vi "remove node name.vi"(8 "error in (no error)":errorcluster, 11 "Data Value Reference in":refnum<data-value>) -> (0 "error out":errorcluster, 3 "Data Value Reference out":refnum<data-value>, 5 "nodes alive":string[](array[string]))   [LabVIEW 2020, in "Publisher Subscriber.lvlib"]
uses:
  Publisher Subscriber.lvlib
  Controls/node dvr data.ctl
  Controls/data cluster.ctl
  Controls/subscription bank ref.ctl
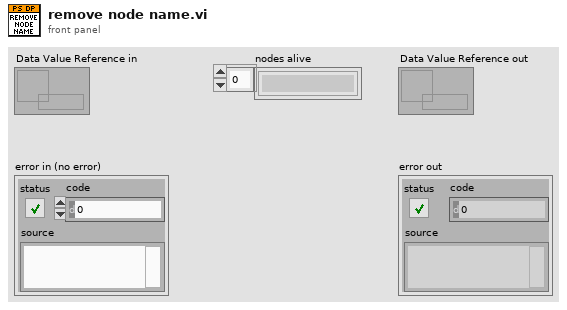
[diagram p1: front panel]
types:
  T1 = typedef "Publisher Subscriber.lvlib/node dvr data.ctl" = cluster{"queue ref":refnum<queue>, "Subscription Bank Ref":refnum<data-value>, "Command":string, "Data":variant, "Subscriptions []":set{string}, "Variables DVR Ref":refnum<data-value>}
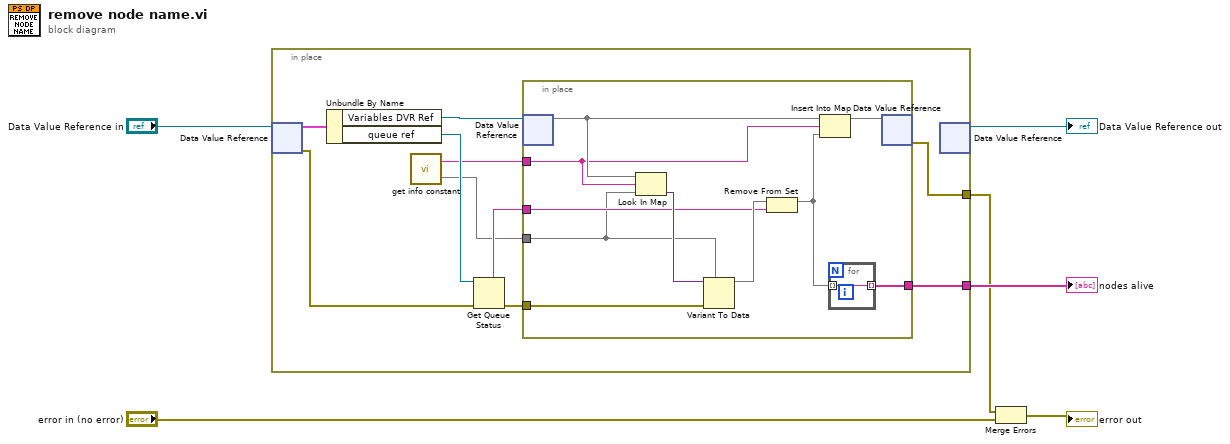
[diagram p0: block diagram]
diagram:
  n1 = in-place {
    in-place-border: [w11] -> w3
    in-place-border: [w10] -> w4
    n2 = in-place-dvr #1("Data Value Reference in") -> (w16:T1, w9:errorcluster)
    n3 = Unbundle By Name(w16) -> ("Variables DVR Ref"=w15:refnum<data-value>, "queue ref"=w14:refnum<queue>)
    n4 = call "get info constant.vi"() -> ("set"=w7:set{string}, "String"=w8:string)  [unwired: 4 in]
    n5 = Get Queue Status(queue=w14, error in (no error)=w9) -> (queue name=w13:string, error out=w12:errorcluster)  [unwired: 1 in, 6 out]
    n6 = in-place {
      in-place-border: w13 -> [w23]
      in-place-border: w8 -> [w22]
      in-place-border: w12 -> [w20]
      in-place-border: [w19] -> w10
      in-place-border: w7 -> [w17]
      n7 = in-place-dvr #2(w15) -> (w26:map{string, variant})  [unwired: 1 out]
      n8 = Look In Map(map=w26, key=w22, default value=w17) -> (value=w25:variant)  [unwired: 1 out]
      n9 = Variant To Data(error in=w20, type=w17, Variant=w25) -> (data=w24:set{string})  [unwired: 1 out]
      n10 = Remove From Set(10:w23, 11:w24) -> (3:w18:set{string})  [unwired: 1 out]
      n11 = Insert Into Map(map in=w26, key=w22, value=w18) -> (map out=w21:map{string, variant})  [unwired: 2 out]
      n12 = for {
        tunnel: [w27] -> w19 mode=indexing
        tunnel: w18 -> [w27] mode=indexing
      }
      n13 = in-place-dvr #2(w21) -> (w11:errorcluster)  [unwired: 1 out]
    }
    n14 = in-place-dvr #1() -> (→"Data Value Reference out":refnum<data-value>)  [unwired: 1 in, 1 out]
  }
  "nodes alive" <- w4
  n15 = Merge Errors(w3, "error in (no error)") -> (→"error out":errorcluster)
